vi "Smooth.vi"(9 "Bit 3":bool, 10 "Bit 2":bool, 11 "Bit 1":bool) -> (2 "Smooth 2":bool)   [LabVIEW 2012]
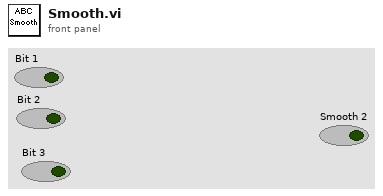
[diagram p1: front panel]
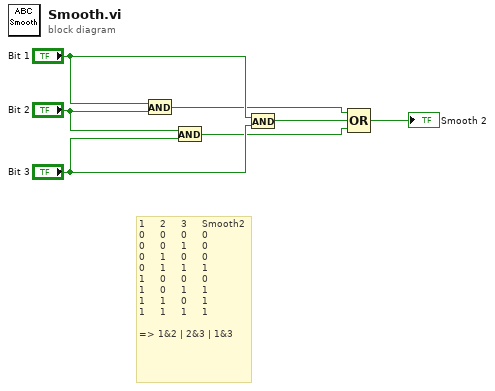
[diagram p0: block diagram]
diagram:
  # "1     2     3     Smooth2\n0     0     0     0\n0     0     1     0\n0     1     0     0\n0     1     1     1\n1     0     0     0\n1     0     1     1\n1     1     0     1\n1     1     1     1\n\n=> 1&2 | 2&3 | 1&3"
  n1 = And(x="Bit 1", y="Bit 2") -> (x .and. y?=w4:bool)
  n2 = And(x="Bit 2", y="Bit 3") -> (x .and. y?=w2:bool)
  n3 = And(x="Bit 1", y="Bit 3") -> (x .and. y?=w3:bool)
  n4 = Compound Arithmetic op=OR(w4, w3, w2) -> (→"Smooth 2":bool)
